vi "Read REST Client.vi"(8 "error in (no error)":errorcluster, 11 "EnVision REST in":refnum<class "EnVision REST.lvclass">) -> (0 "error out":errorcluster, 2 "REST Client.lvlib:REST Client.lvclass":refnum<class "REST Client.lvclass">, 3 "EnVision REST out":refnum<class "EnVision REST.lvclass">)   [LabVIEW 2018, in "EnVision REST.lvlib" / "EnVision REST.lvclass"]
uses:
  EnVision REST.lvclass
  <vilib>/addons/_JKI.lib/REST Client/classes/REST Client/REST Client.lvclass
  EnVision REST.lvclass/EnVision REST.ctl
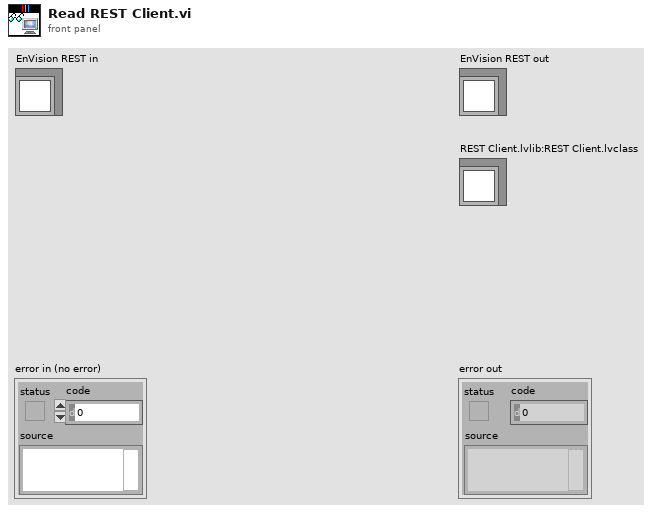
[diagram p1: front panel]
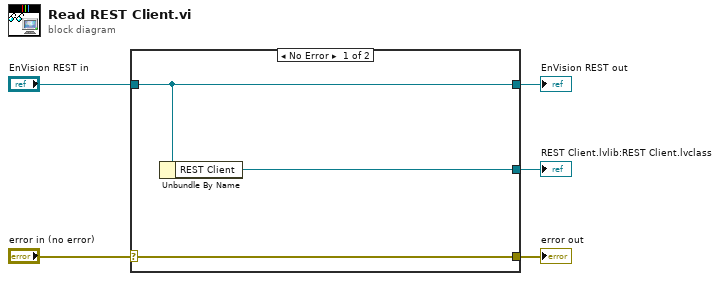
[diagram p0: block diagram]
diagram:
  n1 = case shown="No Error" "error in (no error)" {
    selector: "error in (no error)" -> [w8 w9]
    tunnel: [w8 w9] -> w4
    tunnel: [w7 w10] -> w2
    tunnel: "EnVision REST in" -> [w7 w10]
    tunnel: [w6 _] -> w1
    frame No Error {
      n2 = Unbundle By Name(w7) -> ("REST Client"=w6:refnum<class "REST Client.lvclass">)
    }
    frame Error {
    }
  }
  "error out" <- w4
  "EnVision REST out" <- w2
  "REST Client.lvlib:REST Client.lvclass" <- w1
